vi "Visa Read and Write .vi"() -> ()   [LabVIEW 2016]
uses:
  <vilib>/Instr/_visa.llb/VISA Configure Serial Port (Instr).vi
panel:
  out "x > y?":bool
  out "Gauge":dbl(knob) scale=0.0..5.0
  in  "stop":bool
  in  "VISA resource name":refnum<visa-resource-name>
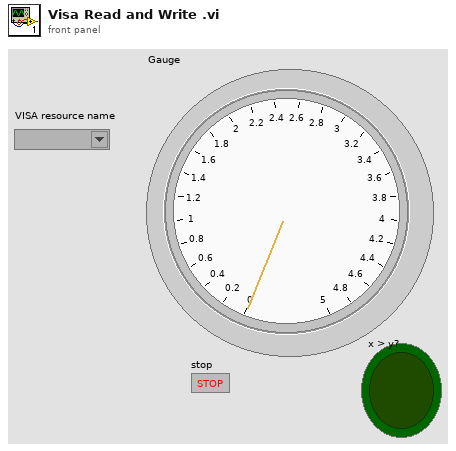
[diagram p1: front panel]
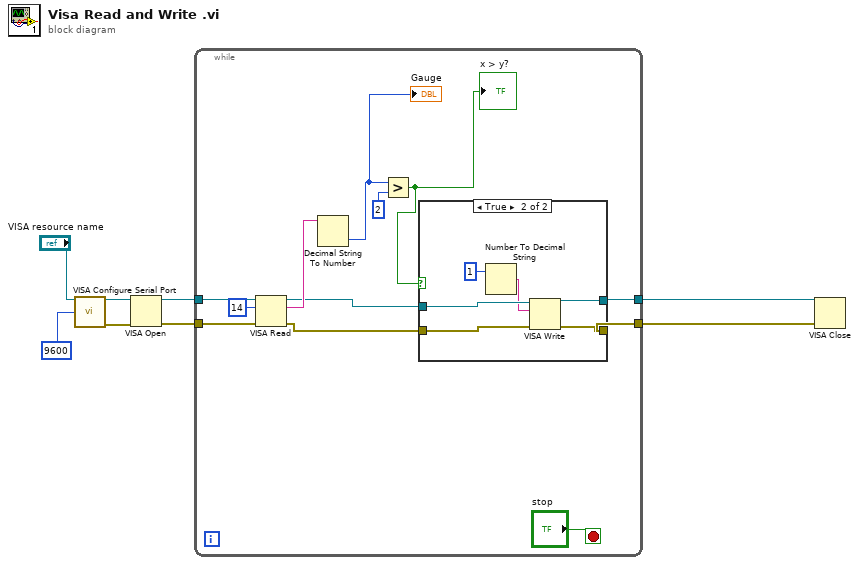
[diagram p0: block diagram]
diagram:
  n1 = call-poly "VISA Configure Serial Port"("VISA resource name"="VISA resource name", "baud rate (9600)"=u32 9600) -> ("VISA resource name out"=w7:refnum<visa-resource-name>, "error out"=w8:errorcluster)  [unwired: 12 in]
  n2 = VISA Open(error in (no error)=w8, VISA resource name=w7) -> (VISA resource name=w6:refnum<visa-resource-name>, error out=w5:errorcluster)  [unwired: 3 in]
  n3 = while {
    tunnel: w6 -> [w20]
    tunnel: w5 -> [w19]
    tunnel: [w10] -> w4
    tunnel: [w9] -> w3
    stop <- "stop" stop-if-true
    n4 = VISA Read(VISA resource name=w20, byte count=u32 14, error in (no error)=w19) -> (VISA resource name out=w12:refnum<visa-resource-name>, read buffer=w18:string, error out=w11:errorcluster)  [unwired: 1 out]
    n5 = Decimal String To Number(string=w18) -> (number=w15:i32)  [unwired: 2 in, 1 out]
    "Gauge" <- w15
    n6 = Greater?(x=w15, y=2 ("x")) -> (0:w13:bool)
    "x > y?" <- w13
    n7 = case shown="True" w13 {
      tunnel: w12 -> [w22 w28]
      tunnel: [w22 w27] -> w9
      tunnel: [w21 w26] -> w10
      tunnel: w11 -> [w21 w25]
      frame False {
      }
      frame True {
        n8 = Number To Decimal String(number=1) -> (decimal integer string=w24:string)  [unwired: 1 in]
        n9 = VISA Write(VISA resource name=w28, write buffer=w24, error in (no error)=w25) -> (VISA resource name out=w27:refnum<visa-resource-name>, error out=w26:errorcluster)  [unwired: 1 out]
      }
    }
  }
  n10 = VISA Close(VISA resource name=w3, error in (no error)=w4) -> ()  [unwired: 1 out]
